vi "onDestroy.vi"(8 "error in (no error)":errorcluster, 11 "MQTT_Base in":refnum<class "MQTT_Base.lvclass">) -> (0 "error out":errorcluster, 3 "MQTT_Base out":refnum<class "MQTT_Base.lvclass">)   [LabVIEW 2013, in "MQTT Server.lvlib" / "MQTT_Base.lvclass"]
uses:
  MQTT_Base.lvclass
  MQTT_Base.lvclass/MQTT_Base.ctl
  Server/Subscription/Subscription.lvclass
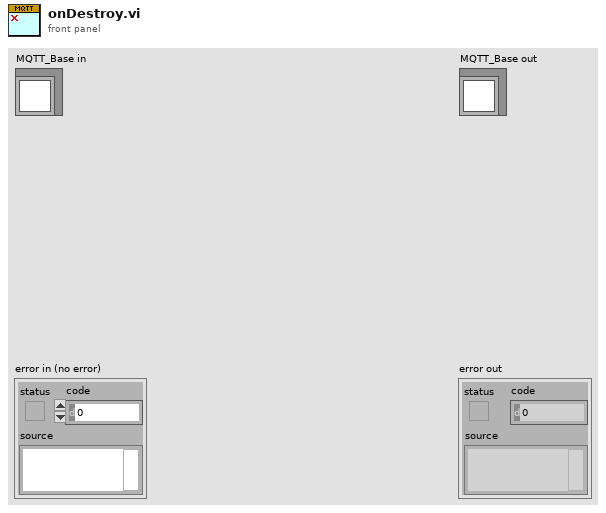
[diagram p1: front panel]
types:
  T1 = typedef "MQTT Server.lvlib/MQTT_Base.lvclass/SessionRef -- cluster.ctl" = cluster{"ClientID":string, "SessionMailbox":refnum<queue>}
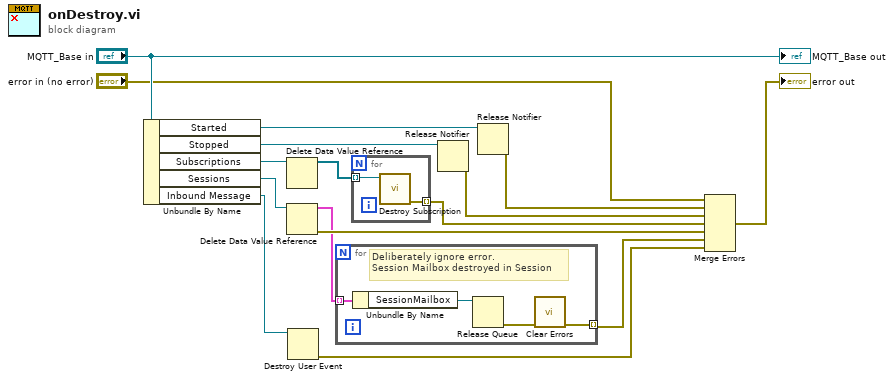
[diagram p0: block diagram]
diagram:
  n1 = Unbundle By Name("MQTT_Base in") -> ("Started"=w8:refnum<notifier>, "Stopped"=w9:refnum<notifier>, "Subscriptions"=w10:refnum<data-value>, "Sessions"=w11:refnum<data-value>, "Inbound Message"=w3:refnum<user-event>)
  n2 = Delete Data Value Reference(data value reference=w10) -> (data value=w12:refnum<class "Subscription.lvclass">[])  [unwired: 1 in, 1 out]
  n3 = Delete Data Value Reference(data value reference=w11) -> (data value=w4:T1[], error out=w14:errorcluster)  [unwired: 1 in]
  n4 = Destroy User Event(user event=w3) -> (error out=w2:errorcluster)  [unwired: 1 in]
  n5 = for {
    tunnel: w4 -> [w20] mode=indexing
    tunnel: [w17] -> w1 mode=indexing
    # "Deliberately ignore error.\nSession Mailbox destroyed in Session"
    n6 = Unbundle By Name(w20) -> ("SessionMailbox"=w19:refnum<queue>)
    n7 = Release Queue(queue=w19) -> (error out=w18:errorcluster)  [unwired: 2 in, 2 out]
    n8 = call <vilib>:"Clear Errors.vi"("error in (no error)"=w18) -> ("error out"=w17:errorcluster)  [unwired: 6 in]
  }
  n9 = for {
    tunnel: w12 -> [w22] mode=indexing
    tunnel: [w21] -> w13 mode=indexing
    n10 = call "Destroy Subscription.vi"("Subscription in"=w22) -> ("error out"=w21:errorcluster)  [unwired: 9 in, 1 out]
  }
  n11 = Release Notifier(notifier=w9) -> (error out=w16:errorcluster)  [unwired: 2 in, 2 out]
  n12 = Release Notifier(notifier=w8) -> (error out=w15:errorcluster)  [unwired: 2 in, 2 out]
  n13 = Merge Errors("error in (no error)", w15, w16, w13, w14, w1, w2) -> (→"error out":errorcluster)
  "MQTT_Base out" <- "MQTT_Base in"
